vi "Convert Pot to Energy.vi"(10 "Initial Voltage (V)":dbl, 11 "Radiation":string) -> (3 "Energy":dbl)   [LabVIEW 2013]
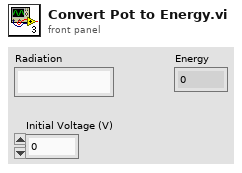
[diagram p1: front panel]
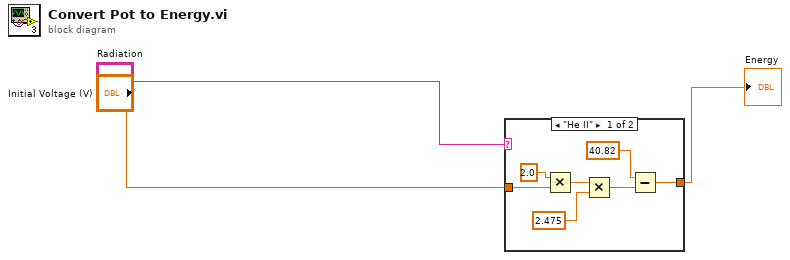
[diagram p0: block diagram]
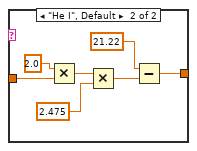
[diagram p2: hidden frame]
diagram:
  n1 = case shown="\"He II\"" "Radiation" {
    tunnel: "Initial Voltage (V)" -> [w8 w17]
    tunnel: [w6 w13] -> w1
    frame "He II" {
      n2 = Multiply(x=2.0, y=w8) -> (x*y=w5:dbl)
      n3 = Multiply(x=w5, y=2.475) -> (x*y=w9:dbl)
      n4 = Subtract(x=40.82, y=w9) -> (x-y=w6:dbl)
    }
    frame "He I", Default {
      n5 = Multiply(x=2.0, y=w17) -> (x*y=w12:dbl)
      n6 = Multiply(x=w12, y=2.475) -> (x*y=w15:dbl)
      n7 = Subtract(x=21.22, y=w15) -> (x-y=w13:dbl)
    }
  }
  "Energy" <- w1
